vi "Destroy.vi"(8 "error in (no error)":errorcluster, 11 "ClientPool in":refnum<class "ClientPool.lvclass">) -> (0 "error out":errorcluster)   [LabVIEW 2020, in "MeasurementLink Measurement Server.lvlib" / "ClientPool.lvclass"]
uses:
  ClientPool.lvclass
  ClientPool.lvclass/ClientPool.ctl
  MeasurementLink Discovery Client/MeasurementLink Discovery Client.lvlib
  MeasurementLink Pin Map Client/MeasurementLink Pin Map Client.lvlib
  MeasurementLink Session Management Client/MeasurementLink Session Management Client.lvlib
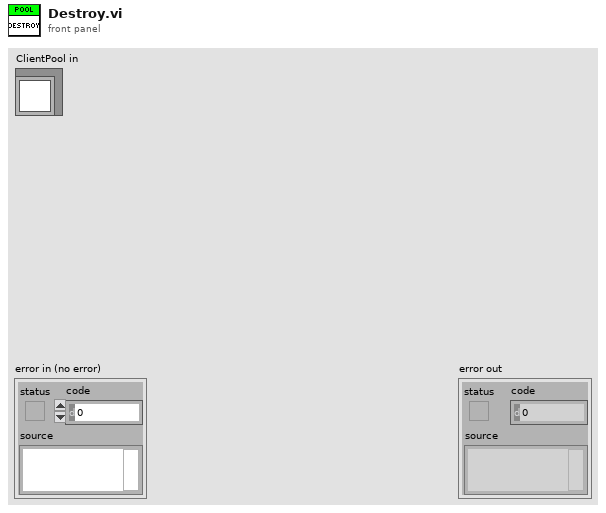
[diagram p1: front panel]
types:
  T1 = typedef "grpc-lvsupport-release.lvlib/grpcId.ctl" = u64
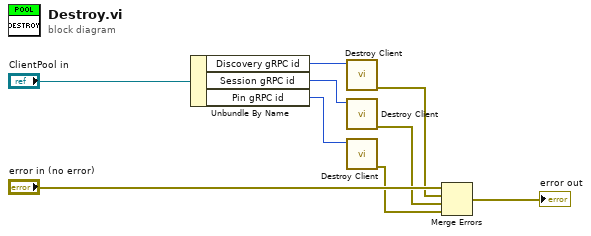
[diagram p0: block diagram]
diagram:
  n1 = Unbundle By Name("ClientPool in") -> ("Discovery gRPC id"=w7:T1, "Session gRPC id"=w6:T1, "Pin gRPC id"=w5:T1)
  n2 = call "Destroy Client.vi"("gRPC ID"=w7) -> ("error out"=w3:errorcluster)  [unwired: 10 in]
  n3 = call "Destroy Client.vi"("gRPC ID"=w6) -> ("error out"=w2:errorcluster)  [unwired: 10 in]
  n4 = call "Destroy Client.vi"("gRPC ID"=w5) -> ("error out"=w1:errorcluster)  [unwired: 10 in]
  n5 = Merge Errors("error in (no error)", w3, w2, w1) -> (→"error out":errorcluster)
